vi "CLD 6 CSV file utility Solution.vi"(8 "Error In":errorcluster, 10 "[Data In]":T1[](array[typedef]), 11 "Read/ Write":T2) -> (0 "Error Out":errorcluster, 3 "[Data Out]":T1[](array[typedef]))   [LabVIEW 2009]
doc: "CLD 6 This VI is a utility that reads the \"CLD CSV File.csv\" file and places the data into the \"CLD Six CSV file data structure.ctl\" data cluster.\n\nTesting Tip:\n\nThere is a Boolean control that can be defaulted to insure the FGV looks for the data file either in the same directory as the FGV (useful for testing) or in the callers directory, if the caller is in a standard CLD test hierarchy, one directory above the subVI directory."
uses:
  CLD 6 CSV file data structure.ctl
  <vilib>/Utility/file.llb/Write To Spreadsheet File (string).vi
  <vilib>/Utility/file.llb/Read From Spreadsheet File (string).vi
  CLD 6 CSV file enum.ctl
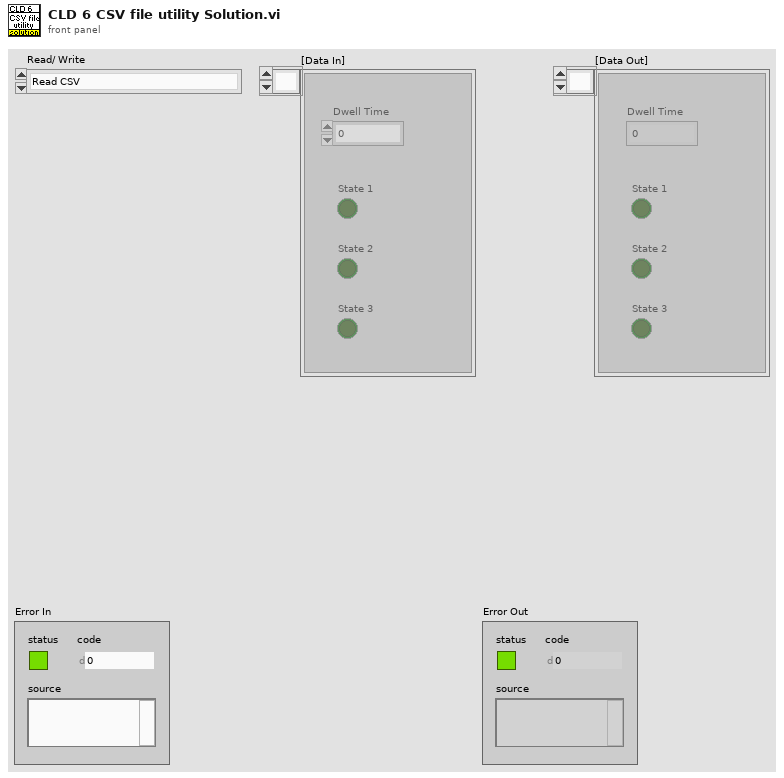
[diagram p1: front panel]
types:
  T1 = typedef "CLD 6 CSV file data structure.ctl" = cluster{"Dwell Time":i32, "State 1":bool, "State 2":bool, "State 3":bool}
  T2 = typedef "CLD 6 CSV file enum.ctl" = enum16{"Read CSV", "Write CSV"}
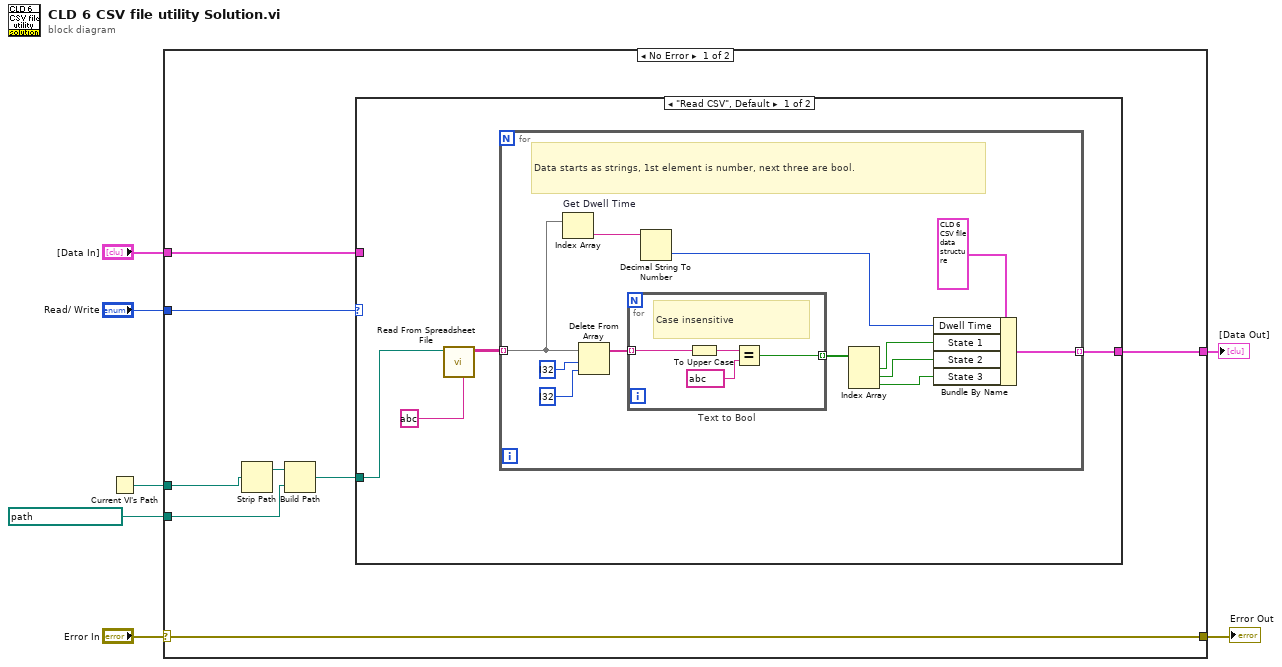
[diagram p0: block diagram]
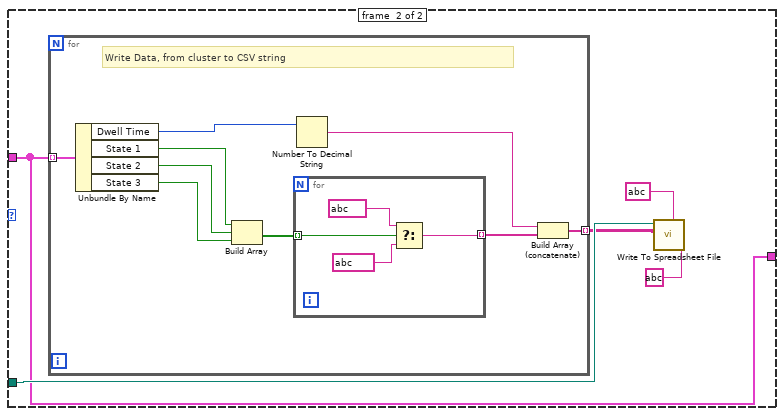
[diagram p2: hidden frame]
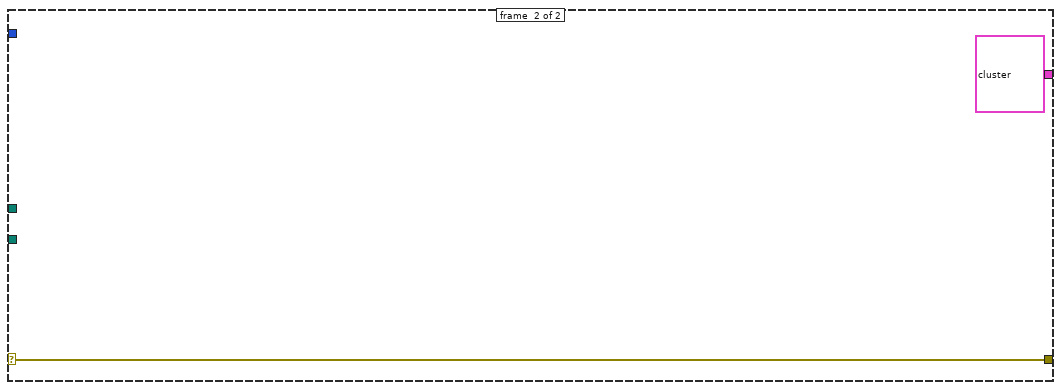
[diagram p3: hidden frame]
diagram:
  n1 = Current VI's Path() -> (path=w5:path)
  n2 = case shown="No Error" "Error In" {
    selector: "Error In" -> [w9 w55]
    tunnel: [w15 T1[] ? ("[Data In]")] -> w7
    tunnel: path ? -> [w14 _]
    tunnel: w5 -> [w13 _]
    tunnel: "Read/ Write" -> [w11 _]
    tunnel: "[Data In]" -> [w10 _]
    tunnel: [w9 w55] -> w1
    frame #0 {
      n3 = Strip Path(path=w13) -> (stripped path=w8:path)  [unwired: 1 out]
      n4 = Build Path(base path=w8, name or relative path=w14) -> (appended path=w12:path)
      n5 = case shown="\"Read CSV\", Default" w11 {
        tunnel: w12 -> [w19 w40]
        tunnel: [w17 w36] -> w15
        tunnel: w10 -> [_ w36]
        frame #0 {
          n6 = call-poly <vilib>:"Read From Spreadsheet File.vi"("delimiter (\\t)"=string ? ("delimiter (\\t)"), "file path (dialog if empty)"=w19) -> ("all rows"=w18:string[][])  [unwired: 5 in, 4 out]
          n7 = for {
            tunnel: w18 -> [w28] mode=indexing
            tunnel: [w31] -> w17 mode=indexing
            # "Data starts as strings, 1st element is number, next three are bool."
            n8 = Index Array "Get Dwell Time"(array=w28) -> (element=w30:string)  [unwired: 1 in]
            n9 = Delete From Array(array=w28, length=i32 ?, index=i32 ?) -> (array with subset deleted=w21:string[])  [unwired: 1 out]
            n10 = for "Text to Bool" {
              tunnel: w21 -> [w35] mode=indexing
              tunnel: [w32] -> w25 mode=indexing
              # "Case insensitive"
              n11 = To Upper Case(1:w35) -> (0:w34:string)
              n12 = Equal?(x=w34, y=string ?) -> (x = y?=w32:bool)
            }
            n13 = Decimal String To Number(string=w30) -> (number=w29:i32)  [unwired: 2 in, 1 out]
            n14 = Index Array(array=w25) -> (element #1=w24:bool, element #2=w23:bool, element #3=w22:bool)  [unwired: 3 in]
            n15 = Bundle By Name(cluster=T1 ? ("CSV File Data Structure"), "Dwell Time"=w29, "State 1"=w24, "State 2"=w23, "State 3"=w22) -> (w31:T1)
          }
        }
        frame #1 {
          n16 = for {
            tunnel: w36 -> [w49] mode=indexing
            tunnel: [w41] -> w38 mode=indexing
            # "Write Data, from cluster to CSV string"
            n17 = Unbundle By Name(w49) -> ("Dwell Time"=w48:i32, "State 1"=w47:bool, "State 2"=w46:bool, "State 3"=w45:bool)
            n18 = Build Array(w47, w46, w45) -> (w44:bool[])
            n19 = for {
              tunnel: w44 -> [w53] mode=indexing
              tunnel: [w50] -> w42 mode=indexing
              n20 = Select(t=string ?, s=w53, f=string ?) -> (s? t:f=w50:string)
            }
            n21 = Number To Decimal String(number=w48) -> (decimal integer string=w43:string)  [unwired: 1 in]
            n22 = Build Array (concatenate)(w43, w42) -> (w41:string[])
          }
          n23 = call-poly <vilib>:"Write To Spreadsheet File.vi"("delimiter (\\t)"=string ? ("delimiter (\\t)"), "format (%s)"=string ?, "2D data"=w38, "file path (dialog if empty)"=w40) -> ()  [unwired: 4 in, 1 out]
        }
      }
    }
    frame #1 {
    }
  }
  "[Data Out]" <- w7
  "Error Out" <- w1
